vi "ProcessPacket.vi"(4 "Message":u8[](array[numeric])) -> ()   [LabVIEW 2015]
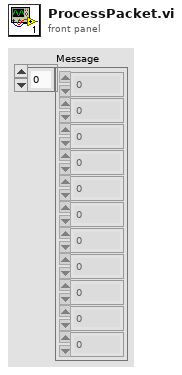
[diagram p1: front panel]
types:
  T1 = typedef "SensorData.ctl" = cluster{"Sensor Id":dbl, "navXPacket":T2, "encoderPacket":T3, "potentiometerPacket":T4, "distanceSensorPacket":T5, "switchPacket":T6, "Sensor Type":T7, "Sensor Status":T8}
  T2 = typedef "navXPacket.ctl" = cluster{"Altitude":dbl, "Barometric Pressure":dbl, "Fused Heading":dbl, "Linear Acceleration Y":dbl, "Linear Acceleration X":dbl, "Temperature":dbl, "Mangnetometer Y":dbl, "Magnetometer X":dbl, "Linear Acceleration Z":dbl}
  T3 = typedef "EncoderPacket.ctl" = cluster{"Encoder Count":dbl, "Encoder Direction":dbl}
  T4 = typedef "PotentiometerPacket.ctl" = cluster{"Angle":dbl}
  T5 = typedef "distanceSensorPacket.ctl" = cluster{"distance":dbl}
  T6 = typedef "switchPacket.ctl" = cluster{"switchValue":bool}
  T7 = typedef "SensorType.ctl" = enum16{"Invalid", "NavX", "Encoder", "Potentiometer", "Distance Sensor", "Switch"}
  T8 = typedef "SensorStatus.ctl" = enum16{"Invalid", "Operational", "Error occurred"}
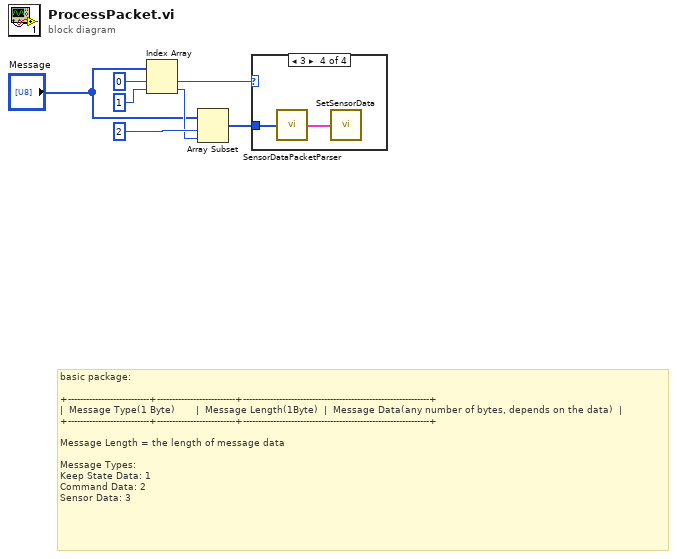
[diagram p0: block diagram]
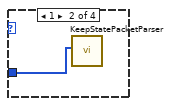
[diagram p3: hidden frame]
diagram:
  # "basic package:\n\n+---------------------------+--------------------------+--------------------------------------------------------------+\n|  Message Type(1 Byte)       |  Message Length(1Byte)\t |  Message Data(any number of bytes, depends on the data)  |\n+---------------------------+--------------------------+--------------------------------------------------------------+\n\nMessage Length = the length of message data\n\nMessage Types:\nKeep State Data: 1\nCommand Data: 2\nSensor Data: 3"
  n1 = Index Array(array="Message", index #1=0 ("index"), index #2=1 ("index")) -> (element #1=w3:u8, element #2=w4:u8)
  n2 = Array Subset(array="Message", index=2, length=w4) -> (w2:u8[])
  n3 = case shown="3" w3 {
    tunnel: w2 -> [_ w8 _ w10]
    frame 0, Default {
    }
    frame 1 {
      n4 = call "KeepStatePacketParser.vi"("Message"=w8) -> ()  [unwired: 11 in]
    }
    frame 2 {
    }
    frame 3 {
      n5 = call "SensorDataPacketParser.vi"("Message"=w10) -> ("Sensor Data"=w9:T1)  [unwired: 4 in]
      n6 = call "SetSensorData.vi"("Sensor Data"=w9) -> ()  [unwired: 5 in]
    }
  }
